vi "Write Log Config Path.vi"(8 "error in (no error)":errorcluster, 10 "Log Config Path":path, 11 "Logger Mananger in":refnum<class "Logger Mananger.lvclass">) -> (0 "error out":errorcluster, 3 "Logger Mananger out":refnum<class "Logger Mananger.lvclass">)   [LabVIEW 2020, in "Logging.lvlib" / "Logger Mananger.lvclass"]
uses:
  Logger Mananger.lvclass
  Logger Mananger.lvclass/Logger Mananger.ctl
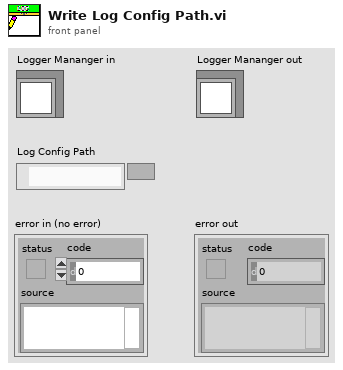
[diagram p1: front panel]
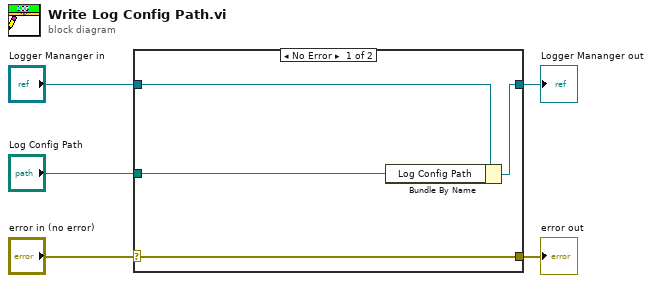
[diagram p0: block diagram]
diagram:
  n1 = case shown="No Error" "error in (no error)" {
    selector: "error in (no error)" -> [w9 w10]
    tunnel: [w9 w10] -> w4
    tunnel: [w7 w11] -> w2
    tunnel: "Logger Mananger in" -> [w8 w11]
    tunnel: "Log Config Path" -> [w6 _]
    frame No Error {
      n2 = Bundle By Name(cluster=w8, "Log Config Path"=w6) -> (w7:refnum<class "Logger Mananger.lvclass">)
    }
    frame Error {
    }
  }
  "error out" <- w4
  "Logger Mananger out" <- w2
